vi "Query S Parameters.vi"(8 "error in (no error)":errorcluster, 10 "Sparameters (string)":string[](array[string]), 11 "VNA-FieldFox in":refnum<class "VNA-FieldFox.lvclass">) -> (0 "error out":errorcluster, 2 "S parameters":T1[](array[typedef]), 3 "VNA-FieldFox out":refnum<class "VNA-FieldFox.lvclass">)   [LabVIEW 2020, in "VNA-FieldFox.lvclass"]
doc: "Queryes the S parameter choosen. It can give single parameter or full 2 to 4 port parameters.\nFor one port S Parameter array only have Sxx.\nFor N ports the S Parameter array hold S11,S12,...,S1N,S21,S22,...,SNN"
uses:
  VNA-FieldFox.lvclass
  C:/Sandbox/RF Bench/Source Code/WiSpry Test Framework/Instruments/Instrument.lvclass
  Controls/Sparameter cluster.ctl
  Instrument.lvclass/Instrument.ctl
  Instrument.lvclass
  <instrlib>/Agilent N99XX Series/Agilent N99XX Series.lvlib
  Vector Network Analyzer.lvclass
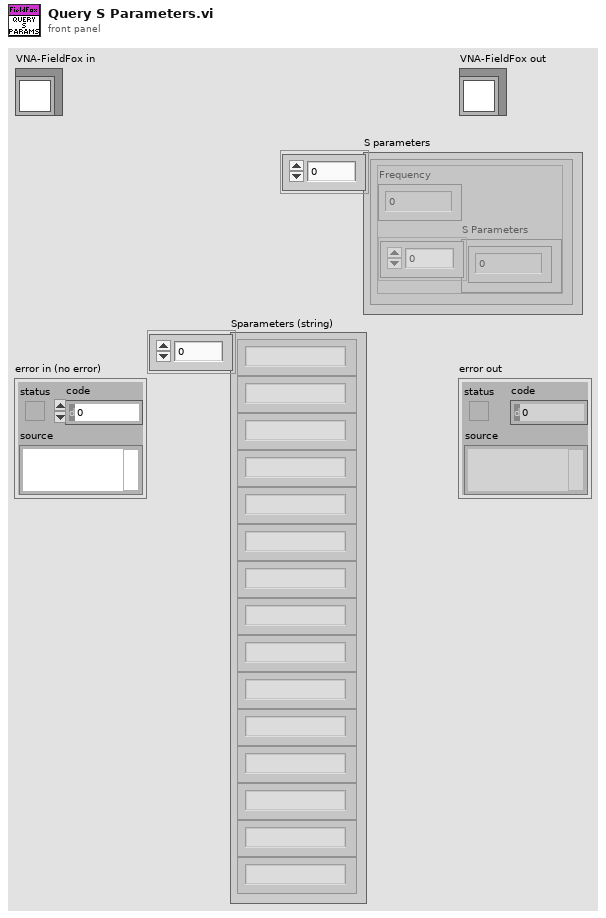
[diagram p1: front panel]
types:
  T1 = typedef "Vector Network Analyzer.lvclass/Sparameter cluster.ctl" = cluster{"Frequency":dbl, "S Parameters":cdb[]}
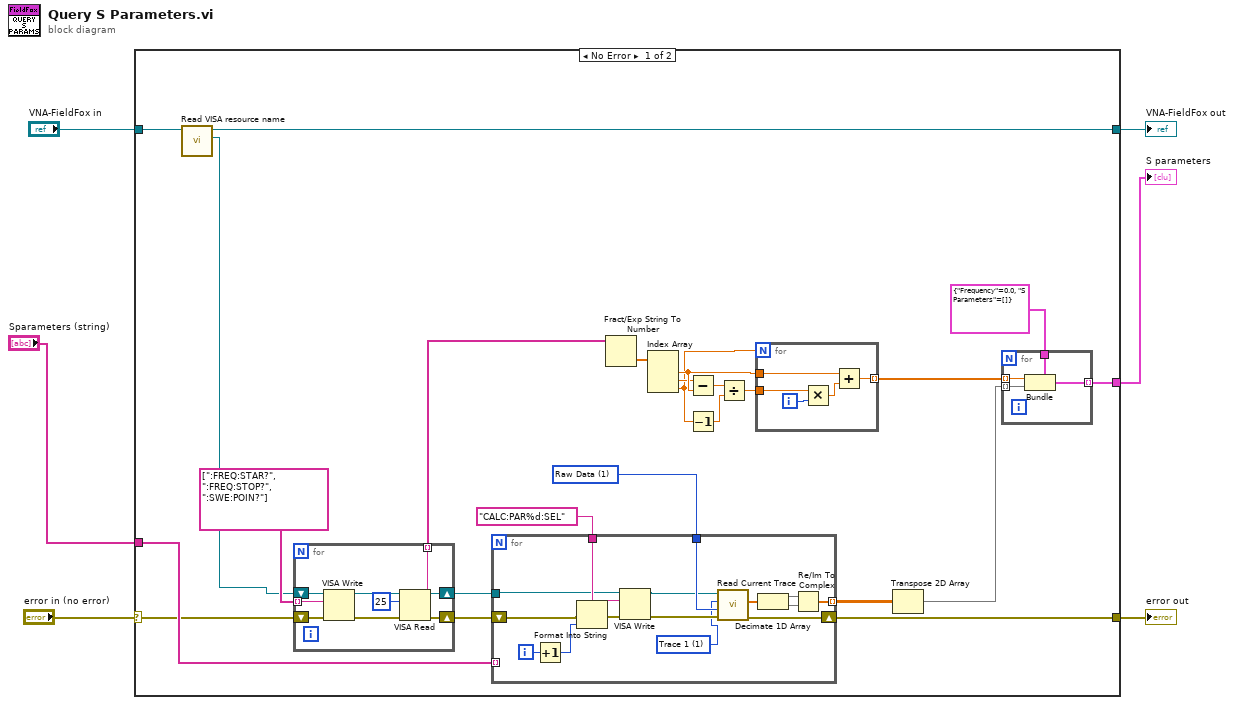
[diagram p0: block diagram]
diagram:
  n1 = case shown="No Error" "error in (no error)" {
    selector: "error in (no error)" -> [w9 w65]
    tunnel: "VNA-FieldFox in" -> [w30 w66]
    tunnel: [w29 w66] -> w4
    tunnel: [w25 _] -> w3
    tunnel: [w24 w65] -> w2
    tunnel: "Sparameters (string)" -> [w23 _]
    frame No Error {
      w28 = 1 items=["Current Format", "Raw Data"] ("Data Type (0: Current Format)")
      n2 = call "Read VISA resource name.vi"("Instrument in"=w30) -> ("VISA resource name"=w8:refnum<visa-resource-name>, "Instrument out"=w29:refnum<class "VNA-FieldFox.lvclass">)  [unwired: 9 in]
      n3 = for {
        tunnel: string[] [":FREQ:STAR?", ":FREQ:STOP?", ":SWE:POIN?"] -> [w39] mode=indexing
        tunnel: [w38] -> w13 mode=indexing
        shift-right: [w42] -> w27
        shift-left: w8 -> [w43]
        shift-right: [w36] -> w22
        shift-left: w9 -> [w37]
        n4 = VISA Write(VISA resource name=w43, write buffer=w39, error in (no error)=w37) -> (VISA resource name out=w44:refnum<visa-resource-name>, error out=w40:errorcluster)  [unwired: 1 out]
        n5 = VISA Read(VISA resource name=w44, byte count=u32 25, error in (no error)=w40) -> (VISA resource name out=w42:refnum<visa-resource-name>, read buffer=w38:string, error out=w36:errorcluster)  [unwired: 1 out]
      }
      n6 = for {
        tunnel: w27 -> [w51]
        tunnel: w28 -> [w63]
        shift-right: [w62] -> w24
        shift-left: w22 -> [w54]
        tunnel: [w58] -> w11 mode=indexing
        tunnel: w23 -> [_] mode=indexing
        tunnel: "CALC:PAR%d:SEL" -> [w55]
        i -> [w64]
        w49 = 1 items=["Trace 1"=1, "Trace 2"=2, "Trace 3"=3, "Trace 4"=4] ("Trace Index (1: Trace 1)")
        n7 = Increment(x=w64) -> (x+1=w50:i32)
        n8 = Format Into String(format string=w55, error in=w54, w50) -> (resulting string=w56:string, error out=w57:errorcluster)  [unwired: 1 in]
        n9 = VISA Write(VISA resource name=w51, write buffer=w56, error in (no error)=w57) -> (VISA resource name out=w52:refnum<visa-resource-name>, error out=w53:errorcluster)  [unwired: 1 out]
        n10 = call <instrlib>:"Read Current Trace.vi"("error in (no error)"=w53, "Data Type (0: Current Format)"=w63, "Trace Index (1: Trace 1)"=w49, "VISA resource name"=w52) -> ("error out"=w62:errorcluster, "Current Trace Data"=w61:dbl[])  [unwired: 3 in, 3 out]
        n11 = Decimate 1D Array(w61) -> (w60:dbl[], w59:dbl[])
        n12 = Re/Im To Complex(1:w59, 2:w60) -> (0:w58:cdb[])
      }
      n13 = Fract/Exp String To Number(string=w13) -> (number=w14:dbl[])  [unwired: 3 in, 1 out]
      n14 = Index Array(array=w14) -> (element #1=w20:dbl, element #2=w19:dbl, element #3=w17:dbl)  [unwired: 3 in]
      n15 = Subtract(x=w19, y=w20) -> (x-y=w18:dbl)
      n16 = Decrement(x=w17) -> (x-1=w16:dbl)
      n17 = Divide(x=w18, y=w16) -> (x/y=w15:dbl)
      n18 = for {
        N: w17 -> [_]
        tunnel: w20 -> [w35]
        tunnel: w15 -> [w33]
        tunnel: [w31] -> w12 mode=indexing
        i -> [w34]
        n19 = Multiply(x=w33, y=w34) -> (x*y=w32:dbl)
        n20 = Add(x=w35, y=w32) -> (x+y=w31:dbl)
      }
      n21 = Transpose 2D Array(2D array=w11) -> (transposed array=w10:cdb[][])
      n22 = for {
        tunnel: T1 {"Frequency"=0.0, "S Parameters"=[]} ("S Parameters") -> [w48]
        tunnel: w12 -> [w47] mode=indexing
        tunnel: w10 -> [w46] mode=indexing
        tunnel: [w45] -> w25 mode=indexing
        n23 = Bundle(cluster=w48, "Frequency"=w47, "S Parameters"=w46) -> (w45:T1)
      }
    }
    frame Error {
    }
  }
  "error out" <- w2
  "VNA-FieldFox out" <- w4
  "S parameters" <- w3
